vi "Build Event from Shots.vi"(10 "Injection.Results":T12 {"Measurements"."Shots"."Results"."Off-Stage Min Volt" format="%#.6g"; "Measurements"."Shots"."Results"."Off-Stage Avg Volt" format="%#.6g"; "Measurements"."Shots"."Results"."Off-Stage Max Volt" format="%#.6g"; "Measurements"."Shots"."Results"."Total Stage Time (us)" format="%#.6g"; "Measurements"."Shots"."Results"."Off-Stage Avg Current" format="%#.6g"; "Measurements"."Shots"."Results"."Total Voltage Pulses" format="%#.6g"; "Measurements"."Shots"."Results"."Off-Stage Min Current" format="%#.6g"; "Measurements"."Shots"."Results"."Off-Stage Max Current" format="%#.6g"}, 11 "Parameters":T1) -> (2 "Injection.Results":T12 {"Measurements"."Shots"."Results"."Off-Stage Min Volt" format="%#.6g"; "Measurements"."Shots"."Results"."Off-Stage Avg Volt" format="%#.6g"; "Measurements"."Shots"."Results"."Off-Stage Max Volt" format="%#.6g"; "Measurements"."Shots"."Results"."Total Stage Time (us)" format="%#.6g"; "Measurements"."Shots"."Results"."Off-Stage Avg Current" format="%#.6g"; "Measurements"."Shots"."Results"."Total Voltage Pulses" format="%#.6g"; "Measurements"."Shots"."Results"."Off-Stage Min Current" format="%#.6g"; "Measurements"."Shots"."Results"."Off-Stage Max Current" format="%#.6g"}, 3 "Parameters":T1)   [LabVIEW 2015, in "Fuel Injector Analysis Addon Engine.lvlib"]
uses:
  Fuel Injector Analysis Addon Engine.lvlib
  Types/Injector Event Data Cluster.ctl
  Controls/Shot Information Control.ctl
  Types/Stage.Measurements.ctl
  Types/Async Parameters.ctl
  Shared/Types/Shot.Parameters.ctl
  Shared/Types/Stage.Parameters.ctl
  Shared/Types/Stage.PullIn.Types.ctl
  Shared/Types/Stage.Transition.Types.ctl
  Shared/Types/Analysis.Channels.Select.ctl
  Shared/Types/Injector info.ctl
  Types/Injector.State.ctl
  <vilib>/NI/NIVS Inline Async API/_Data Access Engine/Data Access Engine/Types/Write.DVR.ctl
  <vilib>/NI/NIVS Inline Async API/_Data Access Engine/Access Type Classes/Write/Write.lvclass
  <vilib>/NI/NIVS Inline Async API/_Data Access Engine/Data Access Engine/Types/Read.DVR.ctl
  <vilib>/NI/NIVS Inline Async API/_Data Access Engine/Access Type Classes/Read/Read.lvclass
  <vilib>/NI Veristand/Custom Device API/Waveform Data Reference.ctl
  <vilib>/NI VeriStand/Custom Device Waveform API/Single Waveform Write (DBL)/Single Waveform Write (DBL).lvclass
  Calculate Hold-In Measurements.vi
  <vilib>/Analysis/baseanly.llb/Mean.vi
  <vilib>/Analysis/baseanly.llb/Mean (DBL).vi
  Calculate Voltage Pulses.vi
  Calculate Hold-In Voltage Measurements.vi
  Shared/Constants.vi
  Shared/Fuel Injector Analysis Addon Shared.lvlib
  <vilib>/NI Veristand/Custom Device API/Custom Device API.lvlib
  <vilib>/NI/NIVS Inline Async API/_Data Access Engine/Data Access Engine/Data Access Engine.lvclass
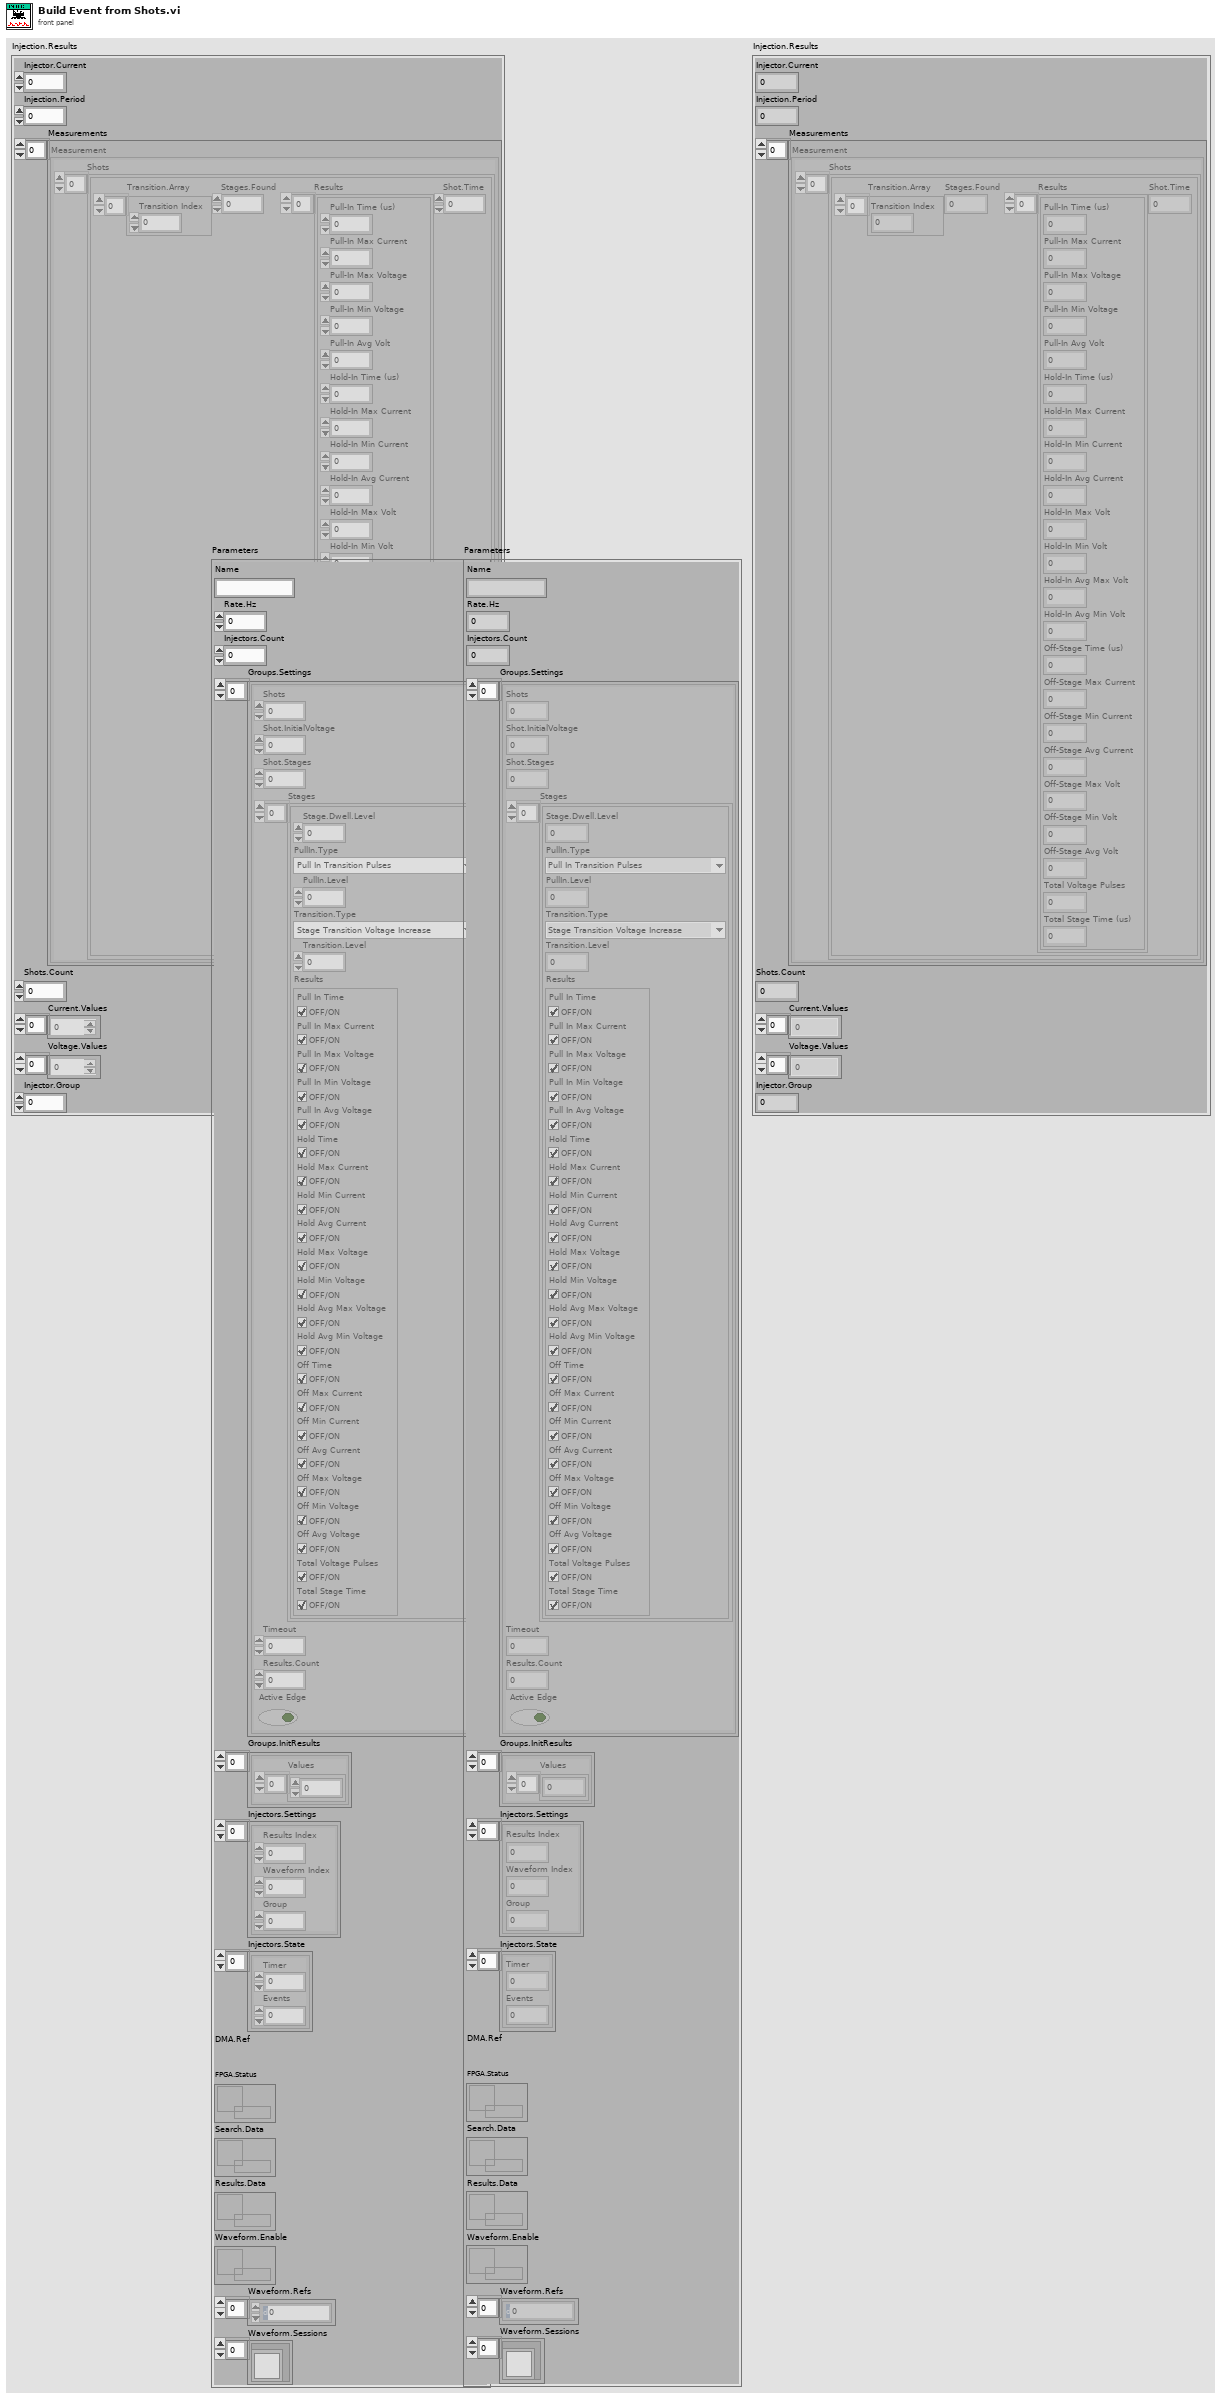
[diagram p1: front panel]
types:
  T1 = typedef "Fuel Injector Analysis Addon Engine.lvlib/Async Parameters.ctl" = cluster{"Name":string, "Rate.Hz":u32, "Injectors.Count":u8, "Groups.Settings":T2[], "Groups.InitResults":cluster{"Values":dbl[]}[], "Injectors.Settings":T7[], "Injectors.State":T8[], "DMA.Ref":refnum<k20>, "FPGA.Status":T9, "Search.Data":T10, "Results.Data":T9, "Waveform.Enable":T10, "Waveform.Refs":T11[], "Waveform.Sessions":refnum<class "Single Waveform Write (DBL).lvclass">[]}
  T2 = typedef "Fuel Injector Analysis Addon Shared.lvlib/Shot.Parameters.ctl" = cluster{"Shots":u32, "Shot.InitialVoltage":dbl, "Shot.Stages":u32, "Stages":T3[], "Timeout":dbl, "Results.Count":i32, "Active Edge":bool}
  T3 = typedef "Fuel Injector Analysis Addon Shared.lvlib/Stage.Parameters.ctl" = cluster{"Stage.Dwell.Level":dbl, "PullIn.Type":T4, "PullIn.Level":dbl, "Transition.Type":T5, "Transition.Level":dbl, "Results":T6}
  T4 = typedef "Fuel Injector Analysis Addon Shared.lvlib/Stage.PullIn.Types.ctl" = enum8{"Pull In Transition Pulses", "Pull In Transition Current Drop"}
  T5 = typedef "Fuel Injector Analysis Addon Shared.lvlib/Stage.Transition.Types.ctl" = enum8{"Stage Transition Inactive Time", "Stage Transition Voltage Increase", "Stage Transition Current Decrease", "Stage Transition Active Time"}
  T6 = typedef "Fuel Injector Analysis Addon Shared.lvlib/Analysis.Channels.Select.ctl" = cluster{"Pull In Time":bool, "Pull In Max Current":bool, "Pull In Max Voltage":bool, "Pull In Min Voltage":bool, "Pull In Avg Voltage":bool, "Hold Time":bool, "Hold Max Current":bool, "Hold Min Current":bool, "Hold Avg Current":bool, "Hold Max Voltage":bool, "Hold Min Voltage":bool, "Hold Avg Max Voltage":bool, "Hold Avg Min Voltage":bool, "Off Time":bool, "Off Max Current":bool, "Off Min Current":bool, "Off Avg Current":bool, "Off Max Voltage":bool, "Off Min Voltage":bool, "Off Avg Voltage":bool, "Total Voltage Pulses":bool, "Total Stage Time":bool}
  T7 = typedef "Fuel Injector Analysis Addon Shared.lvlib/Injector info.ctl" = cluster{"Results Index":i32, "Waveform Index":i32, "Group":u16}
  T8 = typedef "Fuel Injector Analysis Addon Engine.lvlib/Injector.State.ctl" = cluster{"Timer":u32, "Events":u64}
  T9 = typedef "Data Access Engine.lvlib/Data Access Engine.lvclass/Write.DVR.ctl" = refnum<data-value>
  T10 = typedef "Data Access Engine.lvlib/Data Access Engine.lvclass/Read.DVR.ctl" = refnum<data-value>
  T11 = typedef "Custom Device API.lvlib/Waveform Data Reference.ctl" = i32
  T12 = typedef "Fuel Injector Analysis Addon Engine.lvlib/Injector Event Data Cluster.ctl" = cluster{"Injector.Current":i16, "Injection.Period":dbl, "Measurements":cluster{"Shots":T13[]}[], "Shots.Count":i32, "Current.Values":dbl[], "Voltage.Values":dbl[], "Injector.Group":i16}
  T13 = typedef "Fuel Injector Analysis Addon Engine.lvlib/Shot Information Control.ctl" = cluster{"Transition.Array":i32[], "Stages.Found":u16, "Results":T14[], "Shot.Time":dbl}
  T14 = typedef "Fuel Injector Analysis Addon Engine.lvlib/Stage.Measurements.ctl" = cluster{"Pull-In Time (us)":dbl, "Pull-In Max Current":dbl, "Pull-In Max Voltage":dbl, "Pull-In Min Voltage":dbl, "Pull-In Avg Volt":dbl, "Hold-In Time (us)":dbl, "Hold-In Max Current":dbl, "Hold-In Min Current":dbl, "Hold-In Avg Current":dbl, "Hold-In Max Volt":dbl, "Hold-In Min Volt":dbl, "Hold-In Avg Max Volt":dbl, "Hold-In Avg Min Volt":dbl, "Off-Stage Time (us)":dbl, "Off-Stage Max Current":dbl, "Off-Stage Min Current":dbl, "Off-Stage Avg Current":dbl, "Off-Stage Max Volt":dbl, "Off-Stage Min Volt":dbl, "Off-Stage Avg Volt":dbl, "Total Voltage Pulses":dbl, "Total Stage Time (us)":dbl}
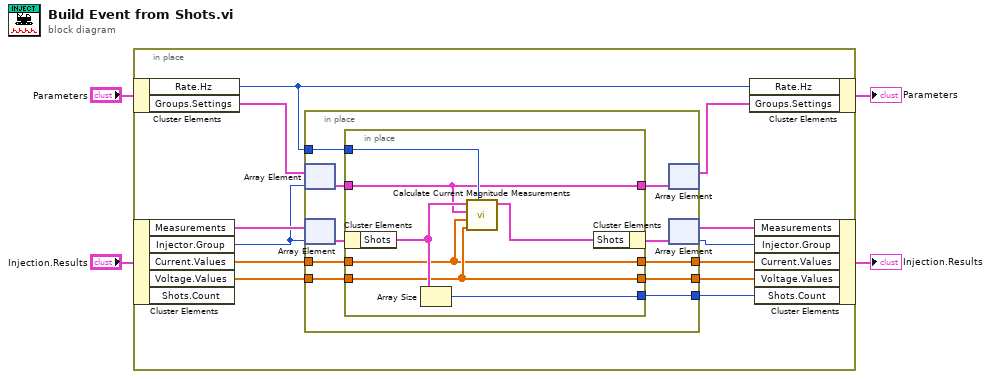
[diagram p0: block diagram]
diagram:
  n1 = in-place {
    n2 = in-place-cluster #1("Parameters") -> ("Rate.Hz"=w16:u32, "Groups.Settings"=w9:T2[])
    n3 = in-place-cluster #2("Injection.Results") -> ("Measurements"=w13:cluster{"Shots":T13[]}[], "Injector.Group"=w12:i16, "Current.Values"=w14:dbl[], "Voltage.Values"=w7:dbl[])  [unwired: 1 out]
    n4 = in-place {
      in-place-border: w16 -> [w26]
      in-place-border: [w25] -> w15
      in-place-border: w14 -> [w24]
      in-place-border: w7 -> [w19]
      in-place-border: [w18] -> w6
      in-place-border: [w17] -> w5
      n5 = in-place-array #3(w9, w12) -> (w22:T2)
      n6 = in-place-array #4(w13, w12) -> (w23:cluster{"Shots":T13[]})
      n7 = in-place {
        in-place-border: w26 -> [w33]
        in-place-border: [w32] -> w25
        in-place-border: w24 -> [w27]
        in-place-border: w19 -> [w28]
        in-place-border: w22 -> [w30]
        in-place-border: [w30] -> w20
        in-place-border: [w28] -> w18
        in-place-border: [w27] -> w17
        n8 = in-place-cluster #5(w23) -> ("Shots"=w31:T13[])
        n9 = Array Size(array=w31) -> (size(s)=w32:i32)
        n10 = call "Calculate Current Magnitude Measurements.vi"("Sample rate (Hz)"=w33, "Voltage Waveform"=w28, "Current Waveform"=w27, "Event.Parameters"=w30, "Shot Info Array"=w31) -> ("Shot Info Array"=w29:T13[])  [unwired: 6 in]
        n11 = in-place-cluster #5("Shots"=w29) -> (w21:cluster{"Shots":T13[]})
      }
      n12 = in-place-array #3(w20) -> (w8:T2[])  [unwired: 1 out]
      n13 = in-place-array #4(w21) -> (w11:cluster{"Shots":T13[]}[], w10:i32)
    }
    n14 = in-place-cluster #1("Rate.Hz"=w16, "Groups.Settings"=w8) -> (→"Parameters":T1)
    n15 = in-place-cluster #2("Measurements"=w11, "Injector.Group"=w10, "Current.Values"=w5, "Voltage.Values"=w6, "Shots.Count"=w15) -> (→"Injection.Results":T12)
  }
